vi "Revision Query.vi"(8 "error in (no error)":errorcluster, 11 "VISA resource name":refnum<visa-resource-name>) -> (0 "error out":errorcluster, 1 "Instrument Firmware Revision":string, 2 "Instrument Driver Revision":string, 3 "VISA resource name out":refnum<visa-resource-name>)   [LabVIEW 2023, in "Keithley DMM6500 DAQ6500 Series.lvlib"]
doc: "Queries the current instrument firmware revision and instrument driver revision.\n\nRefer to the Readme file for detailed driver information including modification history."
uses:
  <instrlib>/Keithley DMM6500 DAQ6500 Series/Keithley DMM6500 DAQ6500 Series.lvlib
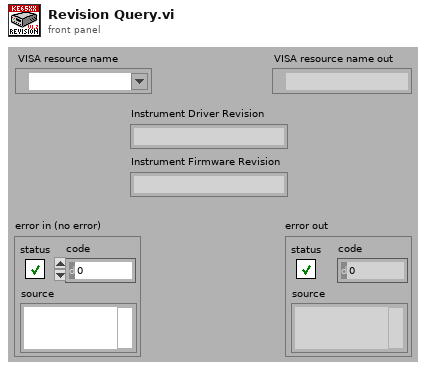
[diagram p1: front panel]
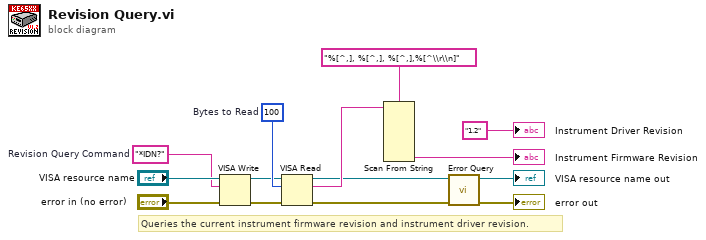
[diagram p0: block diagram]
diagram:
  w9 = "*IDN?"  # Revision Query Command
  w12 = u32 100  # Bytes to Read
  # "Queries the current instrument firmware revision and instrument driver revision."
  n1 = VISA Write(VISA resource name="VISA resource name", write buffer=w9, error in (no error)="error in (no error)") -> (VISA resource name out=w11:refnum<visa-resource-name>, error out=w10:errorcluster)  [unwired: 1 out]
  n2 = VISA Read(VISA resource name=w11, byte count=w12, error in (no error)=w10) -> (VISA resource name out=w5:refnum<visa-resource-name>, read buffer=w8:string, error out=w6:errorcluster)  [unwired: 1 out]
  n3 = Scan From String(format string="%[^,], %[^,], %[^,],%[^\\r\\n]", input string=w8) -> (output 4=→"Instrument Firmware Revision":string)  [unwired: 9 in, 3 out]
  n4 = call <instrlib>:"Error Query.vi"("error in (no error)"=w6, "VISA resource name"=w5) -> ("error out"=→"error out":errorcluster, "VISA resource name out"=→"VISA resource name out":refnum<visa-resource-name>)  [unwired: 6 in, 2 out]
  "Instrument Driver Revision" <- "1.2" ("Instrument Driver Revision")
